vi "Test Relay Control.vi"(8 "error in (no error)":errorcluster, 10 "Connect (False)":bool, 11 "LCM Single-Up MTS Test in":refnum<class "LCM Single-Up MTS Test.lvclass">) -> (0 "error out":errorcluster)   [LabVIEW 2015, in "LCM Single-Up MTS Test.lvclass"]
uses:
  LCM Single-Up MTS Test.lvclass
  CBTF Applications/SmartCast Testing/Main/LCM Single-Up/Application/Application/Class/typedefs/Instrument Selector -- Enum.ctl
  Classes/Instruments/Relay Control/Class/Relay Control.lvclass
  CBTF Applications/SmartCast Testing/Main/LCM Single-Up/Application/Application/Class/LCM Single-Up.lvclass
  Classes/Application/Class/Application.lvclass
  Test Class/Test Class.lvclass
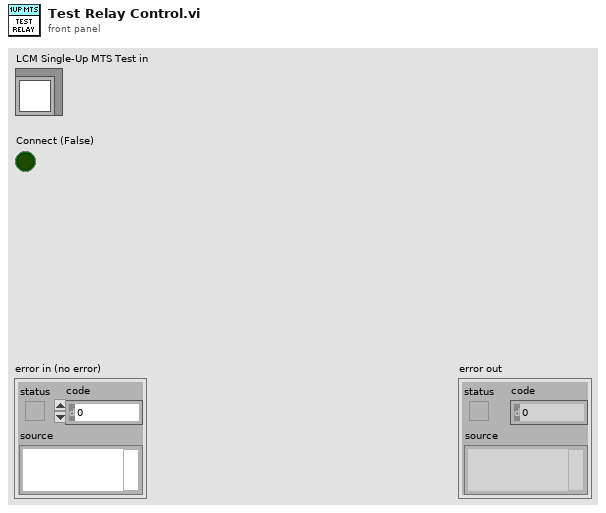
[diagram p1: front panel]
types:
  T1 = typedef "LCM Single-Up.lvlib/LCM Single-Up.lvclass/Instrument Selector -- Enum.ctl" = enum16{"Relay", "MIO Device", "I2C Device", "Thermocouple"}
  T2 = typedef "Application.lvlib/App Properties.lvclass/Class Properties -- Cluster.ctl" = cluster{"UUT Info":T3[], "Test Information":refnum<vi>, "Test Complete Event":refnum<user-event>, "Shop Floor System":refnum<class "Shop Floor System.lvclass">, "Gold Board":refnum<class "Golden Board.lvclass">, "Test Recipe":refnum<class "Test Recipe.lvclass">, "Instruments":refnum<class "Base Class.lvclass">[], "Mode":T4, "Test Results":cluster{"Pass":bool[], "Fail Codes":string[]}, "Station Config":refnum<class "Station Config.lvclass">}
  T3 = typedef "Application.lvlib/App Properties.lvclass/UUT Reference -- Cluster.ctl" = cluster{"Serial Number Reference":refnum<vi>, "Status Message Reference":refnum<vi>}
  T4 = typedef "Application.lvlib/Application.lvclass/Op Mode -- Enum.ctl" = u16
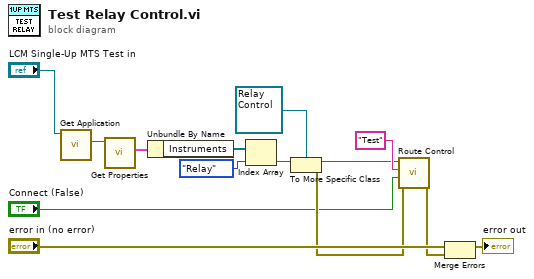
[diagram p0: block diagram]
diagram:
  n1 = call "Get Application.vi"("Test Class in"="LCM Single-Up MTS Test in") -> ("Application.lvlib:Application.lvclass"=w1:refnum<class "Application.lvclass">)  [unwired: 9 in, 1 out]
  n2 = call "Get Properties.vi"("Acrobat Template in"=w1) -> ("Class Properties"=w7:T2)  [unwired: 8 in, 2 out]
  n3 = Unbundle By Name(w7) -> ("Instruments"=w9:refnum<class "Base Class.lvclass">[])
  n4 = Index Array(array=w9, index=Instrument_Selector_--_Enum."Relay" ("Instrument")) -> (element=w8:refnum<class "Base Class.lvclass">)
  n5 = To More Specific Class(target class=refnum<class "Relay Control.lvclass"> refnum ("Relay Control.lvlib:Relay Control.lvclass"), reference=w8) -> (specific class reference=w11:refnum<class "Relay Control.lvclass">, error out=w13:errorcluster)  [unwired: 1 in]
  n6 = call "Route Control.vi"("error in (no error)"=w13, "Connect (False)"="Connect (False)", "Route Name"="Test", "Relay Control in"=w11) -> ("error out"=w3:errorcluster)  [unwired: 6 in, 1 out]
  n7 = Merge Errors("error in (no error)", w3) -> (→"error out":errorcluster)
